vi "Initialize BlackBox Modbus Client TCP.vi"(5 "timeout, ms (300)":u32=300, 6 "station address (255)":u8=255, 7 "protocol (TCP)":enum16{"RTU", "ASCII", "TCP"}(ring)=enum."TCP", 8 "error in (no error)":errorcluster, 9 "port (502)":u16=502, 10 "ip address":string, 11 "PLBB in":refnum<class "PL BlackBox Modbus Client.lvclass">) -> (0 "error out":errorcluster, 3 "PLBB out":refnum<class "PL BlackBox Modbus Client.lvclass">)   [LabVIEW 2015, in "PL BlackBox Modbus Client.lvclass"]
doc: "Initializes TCP connection to BlackBox Modbus server using specified settings."
uses:
  PL BlackBox Modbus Client.lvclass
  <vilib>/plasmapper/PL Modbus Client/PL Modbus Client.lvclass
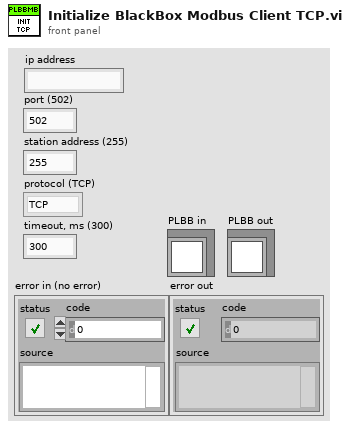
[diagram p1: front panel]
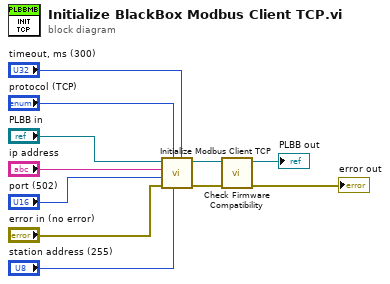
[diagram p0: block diagram]
diagram:
  n1 = call <vilib>:"Initialize Modbus Client TCP.vi"("timeout, ms (300)"="timeout, ms (300)", "station address (255)"="station address (255)", "protocol (TCP)"="protocol (TCP)", "error in (no error)"="error in (no error)", "port (502)"="port (502)", "ip address"="ip address", "MODBUS in"="PLBB in") -> ("error out"=w2:errorcluster, "MODBUS out"=w1:refnum<class "PL BlackBox Modbus Client.lvclass">)  [unwired: 3 in]
  n2 = call-dynamic "Check Firmware Compatibility.vi"("error in (no error)"=w2, "PLBB in"=w1) -> ("error out"=→"error out":errorcluster, "PLBB out"=→"PLBB out":refnum<class "PL BlackBox Modbus Client.lvclass">)  [unwired: 8 in]
